vi "SET_SUPPLY_CHANNEL.vi"(0 "VISA resource name":refnum<visa-resource-name>, 1 "Voltage Level (0.0 V)":dbl format="%.1g", 2 "Enable (OFF)":bool, 5 "Board address":u8, 7 "NChannels":u8, 9 "Channel (0)":u8, 11 "error in (no error)":errorcluster, 12 "Voltage Max (0.0 V)":u16 max=9999, 13 "Current Limit (0.00 uA)":sgl format="%.2g") -> (15 "error out":errorcluster)   [LabVIEW 2012]
uses:
  <instrlib>/CAEN PSM/CAEN PSM.lvlib
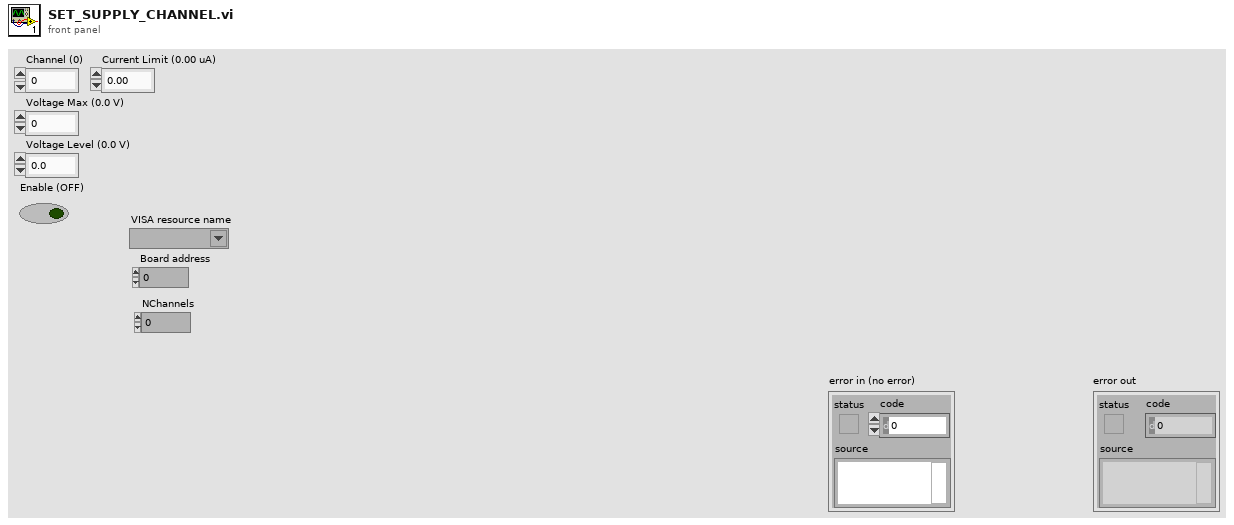
[diagram p1: front panel]
types:
  T1 = cluster{"VISA resource name":refnum<visa-resource-name>, "Board address":u8, "NChannels":u8}
  T2 = typedef "CAEN PSM.lvlib/BoardHandle.ctl" = cluster{"VISA resource name":refnum<visa-resource-name>, "Board address":u8, "NChannels":u8}
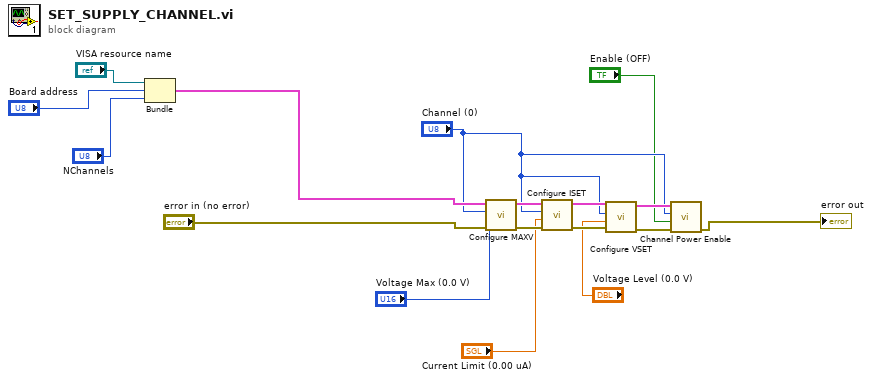
[diagram p0: block diagram]
diagram:
  n1 = Bundle("VISA resource name"="VISA resource name", "Board address"="Board address", "NChannels"="NChannels") -> (w14:T1)  [unwired: 1 in]
  n2 = call <instrlib>:"Configure MAXV.vi"("error in (no error)"="error in (no error)", "Voltage Max (0.0 V)"="Voltage Max (0.0 V)", "Channel (0)"="Channel (0)", "BoardHandle"=w14) -> ("error out"=w9:errorcluster, "BoardHandle out"=w12:T2)  [unwired: 6 in]
  n3 = call <instrlib>:"Configure ISET.vi"("error in (no error)"=w9, "Current Limit (0.00 uA)"="Current Limit (0.00 uA)", "Channel (0)"="Channel (0)", "BoardHandle"=w12) -> ("error out"=w8:errorcluster, "BoardHandle out"=w11:T2)  [unwired: 6 in]
  n4 = call <instrlib>:"Configure VSET.vi"("error in (no error)"=w8, "Voltage Level (0.0 V)"="Voltage Level (0.0 V)", "Channel (0)"="Channel (0)", "BoardHandle"=w11) -> ("error out"=w7:errorcluster, "BoardHandle out"=w10:T2)  [unwired: 6 in]
  n5 = call <instrlib>:"Channel Power Enable.vi"("error in (no error)"=w7, "Enable (OFF)"="Enable (OFF)", "Channel (0)"="Channel (0)", "BoardHandle"=w10) -> ("error out"=→"error out":errorcluster)  [unwired: 6 in, 1 out]
